vi "Move array element up or down.vi"(7 "Action":enum16{"Move Up", "Move Down"}(ring), 10 "index":u16, 11 "Array In":variant[](array[variant])) -> (3 "Array Out":variant[](array[variant]))   [LabVIEW 2023]
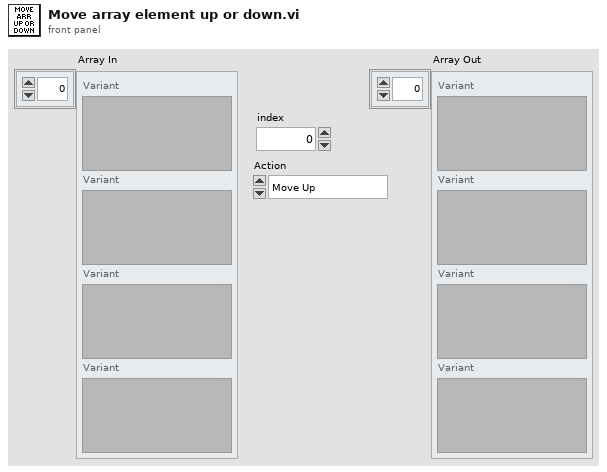
[diagram p1: front panel]
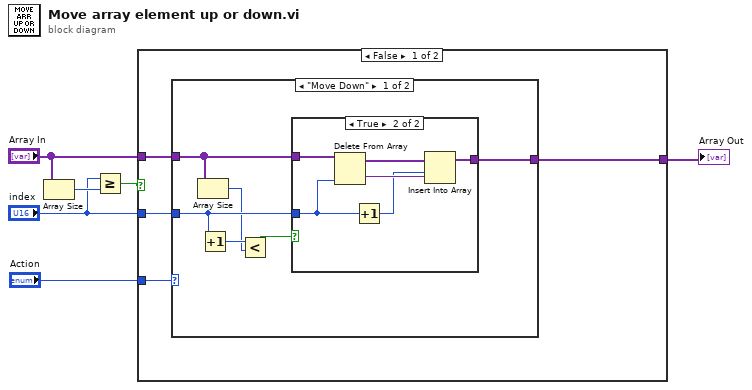
[diagram p0: block diagram]
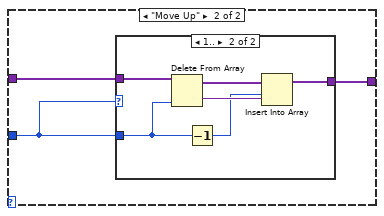
[diagram p3: hidden frame]
diagram:
  n1 = Array Size(array="Array In") -> (size(s)=w4:i32)
  n2 = Greater Or Equal?(x="index", y=w4) -> (x >= y?=w2:bool)
  n3 = case shown="False" w2 {
    tunnel: "Action" -> [w10 _]
    tunnel: "Array In" -> [w9 w34]
    tunnel: "index" -> [w8 _]
    tunnel: [w7 w34] -> w1
    frame False {
      n4 = case shown="\"Move Down\"" w10 {
        tunnel: w9 -> [w15 w26]
        tunnel: w8 -> [w14 w24]
        tunnel: [w16 w25] -> w7
        frame "Move Down" {
          n5 = Array Size(array=w15) -> (size(s)=w12:i32)
          n6 = Increment(x=w14) -> (x+1=w13:u16)
          n7 = Less?(x=w13, y=w12) -> (x < y?=w11:bool)
          n8 = case shown="True" w11 {
            tunnel: [w17 w21] -> w16
            tunnel: w15 -> [w17 w19]
            tunnel: w14 -> [_ w18]
            frame False {
            }
            frame True {
              n9 = Delete From Array(array=w19, index=w18) -> (deleted portion=w22:variant, array with subset deleted=w23:variant[])  [unwired: 1 in]
              n10 = Increment(x=w18) -> (x+1=w20:u16)
              n11 = Insert Into Array(array=w23, index=w20, new element=w22) -> (w21:variant[])
            }
          }
        }
        frame "Move Up" {
          n12 = case shown="1.." w24 {
            tunnel: w26 -> [w27 w33]
            tunnel: [w27 w30] -> w25
            tunnel: w24 -> [_ w29]
            frame 0, Default {
            }
            frame 1.. {
              n13 = Delete From Array(array=w33, index=w29) -> (deleted portion=w31:variant, array with subset deleted=w32:variant[])  [unwired: 1 in]
              n14 = Decrement(x=w29) -> (x-1=w28:u16)
              n15 = Insert Into Array(array=w32, index=w28, new element=w31) -> (w30:variant[])
            }
          }
        }
      }
    }
    frame True {
    }
  }
  "Array Out" <- w1
